vi "Get_measurement_samplingdata.vi"(0 "SPU":refnum<k24>, 1 "STSProcess.PDLSTS":refnum<k24>, 5 "Meas_monitor_struct":refnum<k24>[](array[refnum]), 7 "MPM":refnum<k24>[](array[refnum]), 9 "Data_struct":refnum<k24>[](array[refnum]), 11 "错误输入（无错误）":errorcluster, 12 "SweepCount":i32, 13 "SOP":i32) -> (15 "error out":errorcluster)   [LabVIEW 2017]
doc: "Get logging measurement data & add in"
uses:
  D:/test/PDLSTS/LV_PDL_Sample/DLL/STSProcess.dll
  DLL/STSProcess.dll
  D:/test/PDLSTS/LV_PDL_Sample/DLL/InstrumentDLL.dll
  DLL/InstrumentDLL.dll
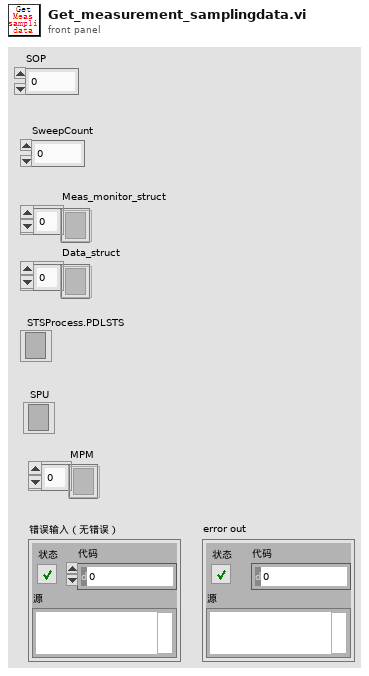
[diagram p1: front panel]
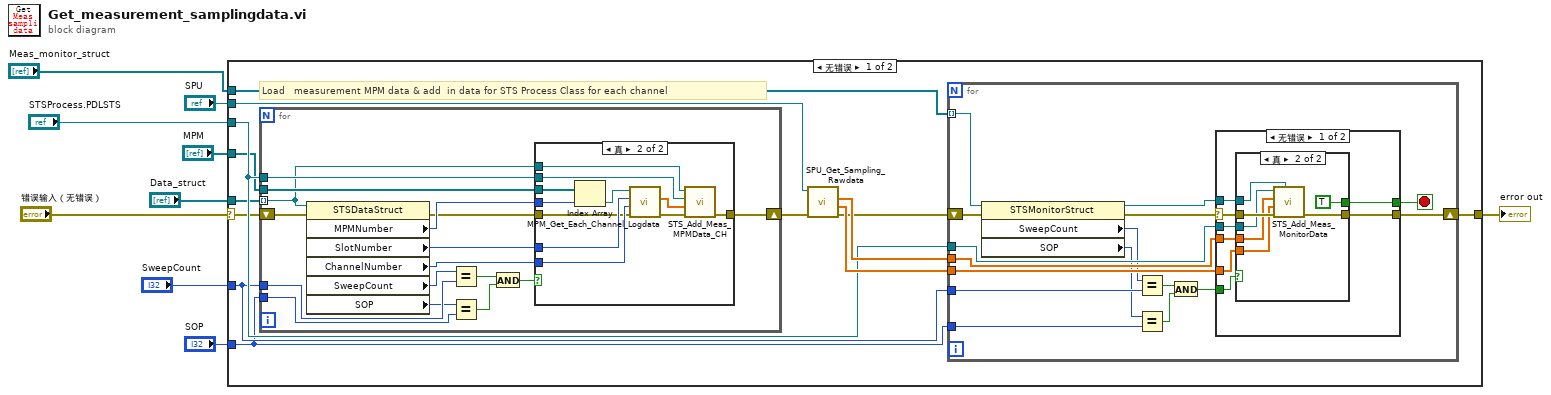
[diagram p0: block diagram]
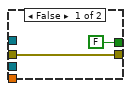
[diagram p2: hidden frame]
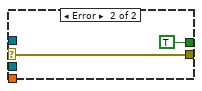
[diagram p3: hidden frame]
diagram:
  n1 = case shown="无错误" "错误输入（无错误）" {
    selector: "错误输入（无错误）" -> [w13 w86]
    tunnel: "STSProcess.PDLSTS" -> [w20 _]
    tunnel: "Meas_monitor_struct" -> [w19 _]
    tunnel: "SPU" -> [w18 _]
    tunnel: "MPM" -> [w16 _]
    tunnel: "Data_struct" -> [w15 _]
    tunnel: [w14 w86] -> w6
    tunnel: "SweepCount" -> [w12 _]
    tunnel: "SOP" -> [w10 _]
    frame No Error {
      # "Load　measurement MPM data & add  in data for STS Process Class for each channel"
      n2 = for {
        tunnel: w15 -> [w65] mode=indexing
        tunnel: w16 -> [w71]
        tunnel: w20 -> [w66]
        tunnel: w12 -> [w63]
        shift-right: [w67] -> w17
        shift-left: w13 -> [w68]
        tunnel: w10 -> [w61]
        n3 = property on="属性节点" class="STSDataStruct"(reference=w65, error in=w68) -> (error out=w69:errorcluster, "MPMNumber"=w70:i32, "SlotNumber"=w73:i32, "ChannelNumber"=w72:i32, "SweepCount"=w64:i32, "SOP"=w62:i32)  [unwired: 1 out]
        n4 = Equal?(x=w64, y=w63) -> (x = y?=w60:bool)
        n5 = Equal?(x=w62, y=w61) -> (x = y?=w59:bool)
        n6 = And(x=w60, y=w59) -> (x .and. y?=w58:bool)
        n7 = case shown="真" w58 {
          tunnel: w73 -> [_ w85]
          tunnel: w72 -> [_ w84]
          tunnel: w71 -> [_ w83]
          tunnel: w70 -> [_ w82]
          tunnel: w69 -> [w74 w81]
          tunnel: [w74 w79] -> w67
          tunnel: w66 -> [_ w76]
          tunnel: w65 -> [_ w75]
          frame False {
          }
          frame True {
            n8 = Index Array(array=w83, index=w82) -> (element=w80:refnum<k24>)
            n9 = call "MPM_Get_Each_Channel_Logdata.vi"("error in (no error)"=w81, "channelNumber"=w84, "moduleNumber"=w85, ".NET Reference in"=w80) -> ("error out"=w78:errorcluster, "data out"=w77:sgl[])  [unwired: 5 in, 1 out]
            n10 = call "STS_Add_Meas_MPMData_CH.vi"("错误输入（无错误）"=w78, "data"=w77, "STSProcess.PDLSTS"=w76, ".NET引用句柄输入"=w75) -> ("错误输出"=w79:errorcluster)  [unwired: 6 in, 1 out]
          }
        }
      }
      n11 = call "SPU_Get_Sampling_Rawdata.vi"("错误输入（无错误）"=w17, "SPU"=w18) -> ("error out"=w11:errorcluster, "monitor"=w22:sgl[], "trigger"=w21:sgl[])  [unwired: 5 in, 1 out]
      n12 = for {
        tunnel: w19 -> [w34] mode=indexing
        tunnel: w20 -> [w38]
        tunnel: w21 -> [w37]
        tunnel: w22 -> [w36]
        shift-right: [w35] -> w14
        shift-left: w11 -> [w30]
        tunnel: w12 -> [w32]
        tunnel: w10 -> [w27]
        stop <- w23 stop-if-true
        n13 = property on="属性节点" class="STSMonitorStruct"(reference=w34, error in=w30) -> (reference out=w31:refnum<k24>, error out=w29:errorcluster, "SweepCount"=w33:i32, "SOP"=w28:i32)
        n14 = Equal?(x=w33, y=w32) -> (x = y?=w26:bool)
        n15 = Equal?(x=w28, y=w27) -> (x = y?=w25:bool)
        n16 = And(x=w26, y=w25) -> (x .and. y?=w24:bool)
        n17 = case shown="无错误" w29 {
          selector: w29 -> [w45 w57]
          tunnel: w38 -> [w44 _]
          tunnel: w31 -> [w41 _]
          tunnel: w37 -> [w43 _]
          tunnel: w36 -> [w42 _]
          tunnel: [w46 w57] -> w35
          tunnel: w24 -> [w40 _]
          tunnel: [w39 TRUE] -> w23
          frame No Error {
            n18 = case shown="真" w40 {
              tunnel: [w48 w55] -> w46
              tunnel: w45 -> [w48 w54]
              tunnel: w44 -> [_ w53]
              tunnel: w43 -> [_ w52]
              tunnel: w42 -> [_ w51]
              tunnel: w41 -> [_ w50]
              tunnel: [FALSE TRUE] -> w39
              frame False {
              }
              frame True {
                n19 = call "STS_Add_Meas_MonitorData.vi"("setting"=w50, "错误输入（无错误）"=w54, "monitorData"=w51, "triggerIndex"=w52, "STSProcess.PDLSTS"=w53) -> ("错误输出"=w55:errorcluster)  [unwired: 5 in, 1 out]
              }
            }
          }
          frame Error {
          }
        }
      }
    }
    frame Error {
    }
  }
  "error out" <- w6
